vi "Flash Get Cooler Status.vi"(8 "error in (no error)":errorcluster, 11 "Orca-Flash 4.0 V2 in":refnum<class "Orca-Flash 4.0 V2.lvclass">) -> (0 "error out":errorcluster, 3 "Orca-Flash 4.0 V2 out":refnum<class "Orca-Flash 4.0 V2.lvclass">)   [LabVIEW 2015]
uses:
  Resources/GLOBAL/GLOBAL General Properties.vi
  Orca-Flash 4.0 V2.lvclass
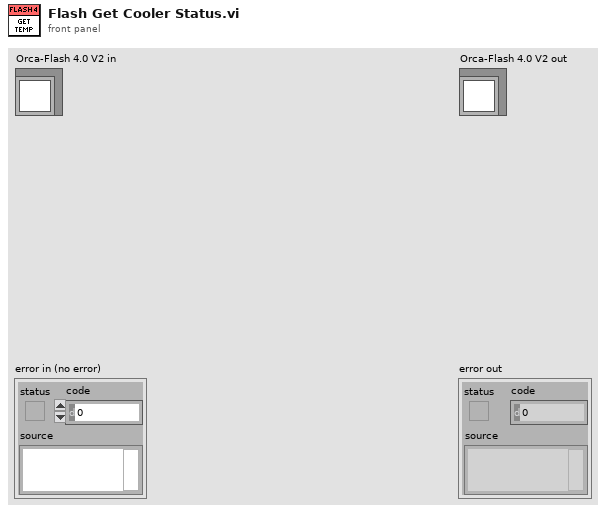
[diagram p1: front panel]
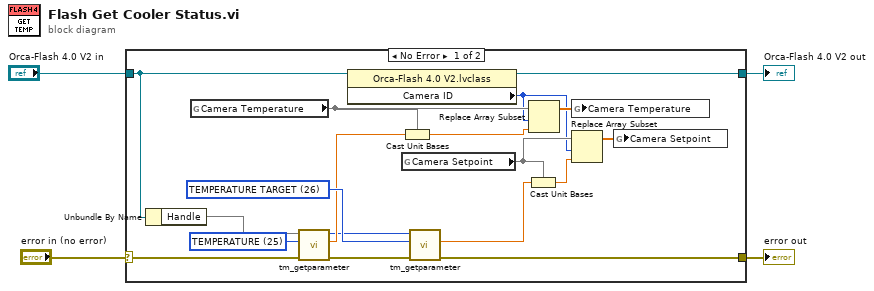
[diagram p0: block diagram]
diagram:
  n1 = case shown="No Error" "error in (no error)" {
    selector: "error in (no error)" -> [w21 w24]
    tunnel: [w17 w24] -> w3
    tunnel: [w15 w23] -> w1
    tunnel: "Orca-Flash 4.0 V2 in" -> [w16 w23]
    frame No Error {
      w19 = u32 26 items=["BINNING"=1, "BITS PER CHANNEL"=2, "ACTIVE VIEW INDEX"=3, "CCD MODE"=4, "SENSOR MODE"=5, "READOUT MODE"=6, "EXPOSURE TIME"=7, "CONTRAST GAIN"=8, "CONTRAST OFFSET"=9, "LIGHT MODE"=10, "SENSITIVITY"=11, "WHITE BALANCE"=12, "PHOTON IMAGING MODE"=13, "HIGH DYNAMIC RANGE MODE"=14, "TRIGGER SOURCE"=15, "TRIGGER ACTIVE"=16, "TRIGGER MODE"=17, "TRIGGER POLARITY"=18, "TRIGGER GLOBAL EXPOSURE"=19, "FIRST TRIGGER BEHAVIOR"=20, "TRIGGER TIMES"=21, "OUTPUT TRIGGER POLARITY"=22, "OUTPUT TRIGGER DELAY"=23, "OUTPUT TRIGGER PERIOD"=24, "TEMPERATURE"=25, "TEMPERATURE TARGET"=26, "SENSOR COOLER FAN"=27, "MECHANICAL SHUTTER"=28, "BACK FOCUS POSITION"=29, "FRAMEBUNDLE MODE"=30, "FRAMEBUNDLE NUMBER"=31, "LINEBUNDLE HEIGHT"=32, "TRIGGER CONNECTOR"=33, "IMAGE PIXEL TYPE"=34, "OUTPUT TRIGGER KIND"=35, "READOUT DIRECTION"=36, "CHANNEL SYNC"=37] ("Parameter")
      w20 = u32 25 items=["BINNING"=1, "BITS PER CHANNEL"=2, "ACTIVE VIEW INDEX"=3, "CCD MODE"=4, "SENSOR MODE"=5, "READOUT MODE"=6, "EXPOSURE TIME"=7, "CONTRAST GAIN"=8, "CONTRAST OFFSET"=9, "LIGHT MODE"=10, "SENSITIVITY"=11, "WHITE BALANCE"=12, "PHOTON IMAGING MODE"=13, "HIGH DYNAMIC RANGE MODE"=14, "TRIGGER SOURCE"=15, "TRIGGER ACTIVE"=16, "TRIGGER MODE"=17, "TRIGGER POLARITY"=18, "TRIGGER GLOBAL EXPOSURE"=19, "FIRST TRIGGER BEHAVIOR"=20, "TRIGGER TIMES"=21, "OUTPUT TRIGGER POLARITY"=22, "OUTPUT TRIGGER DELAY"=23, "OUTPUT TRIGGER PERIOD"=24, "TEMPERATURE"=25, "TEMPERATURE TARGET"=26, "SENSOR COOLER FAN"=27, "MECHANICAL SHUTTER"=28, "BACK FOCUS POSITION"=29, "FRAMEBUNDLE MODE"=30, "FRAMEBUNDLE NUMBER"=31, "LINEBUNDLE HEIGHT"=32, "TRIGGER CONNECTOR"=33, "IMAGE PIXEL TYPE"=34, "OUTPUT TRIGGER KIND"=35, "READOUT DIRECTION"=36, "CHANNEL SYNC"=37] ("Parameter")
      n2 = Unbundle By Name(w16) -> ("Handle"=w22)
      n3 = global read "GLOBAL General Properties.vi" "Camera Temperature"() -> (w12)
      n4 = call <userlib>:"tm_getparameter.vi"("error in (no error)"=w21, "Parameter"=w20, "Handle in"=w22) -> ("error out"=w18:errorcluster, "Value out"=w13:dbl, "Handle out"=w5:u32)  [unwired: 6 in]
      n5 = property class="Orca-Flash 4.0 V2.lvclass"(reference=w16) -> (reference out=w15:refnum<class "Orca-Flash 4.0 V2.lvclass">, "Camera ID"=w7:i32)  [unwired: 1 in, 1 out]
      n6 = Cast Unit Bases(0:w13, 1:w12) -> (2:w11:dbl)
      n7 = global read "GLOBAL General Properties.vi" "Camera Setpoint"() -> (w9)
      n8 = call <userlib>:"tm_getparameter.vi"("error in (no error)"=w18, "Parameter"=w19, "Handle in"=w5) -> ("error out"=w17:errorcluster, "Value out"=w6:dbl)  [unwired: 6 in, 1 out]
      n9 = Cast Unit Bases(0:w6, 1:w9) -> (2:w10:dbl)
      n10 = Replace Array Subset(array=w12, new element=w11, index=w7) -> (w14:dbl[])
      n11 = global write "GLOBAL General Properties.vi" "Camera Temperature"(w14) -> ()
      n12 = Replace Array Subset(array=w9, new element=w10, index=w7) -> (w8:dbl[])
      n13 = global write "GLOBAL General Properties.vi" "Camera Setpoint"(w8) -> ()
    }
    frame Error {
    }
  }
  "error out" <- w3
  "Orca-Flash 4.0 V2 out" <- w1
